vi "simx Synchronous Trigger.vi"(8 "error in (no error)":errorcluster, 11 "clientID":i32) -> (0 "error out":errorcluster, 3 "function return":i32)   [LabVIEW 2019, in "PXL_V-REP.lvlib"]
doc: "EXTAPI_DLLEXPORT simxInt simxSynchronousTrigger(simxInt clientID);"
uses:
  PXL_V-REP.lvlib
  <userlib>/V-REP/remoteApi.dll
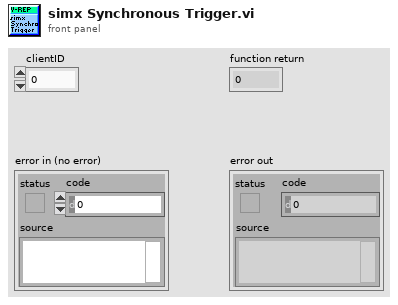
[diagram p1: front panel]
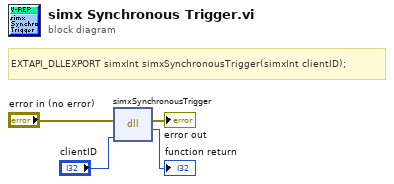
[diagram p0: block diagram]
diagram:
  # "EXTAPI_DLLEXPORT simxInt simxSynchronousTrigger(simxInt clientID);"
  n1 = dll-call lib="C:/Program Files (x86)/National Instruments/LabVIEW 2019/user.lib/V-REP/remoteApi.*" fn="simxSynchronousTrigger"(error in="error in (no error)", "clientID"="clientID") -> (error out=→"error out":errorcluster, →"function return":i32)  [unwired: 3 in, 1 out]
